vi "real time timestamp check.vi"() -> ()   [LabVIEW 2012]
uses:
  <vilib>/Utility/miscctls.llb/LVDateTimeRec.ctl
panel:
  out "epoch delta":ext format="%#_16f"
  out "unix time":ext format="%#_16f"
  out "extended precision float":ext format="%#_16f"
  out "date time rec":T1
  in  "stop":bool
  out "date/time string":string
  out "current time":timestamp
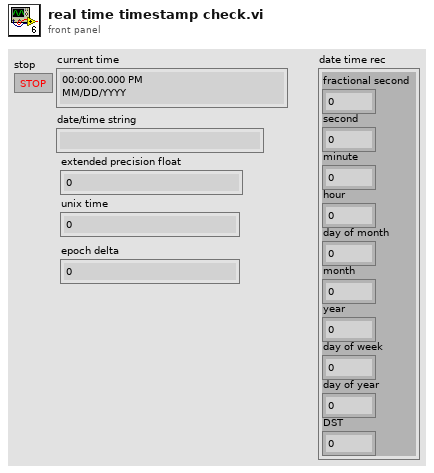
[diagram p1: front panel]
types:
  T1 = typedef "LVDateTimeRec.ctl" = cluster{"fractional second":dbl, "second":i32, "minute":i32, "hour":i32, "day of month":i32, "month":i32, "year":i32, "day of week":i32, "day of year":i32, "DST":i32}
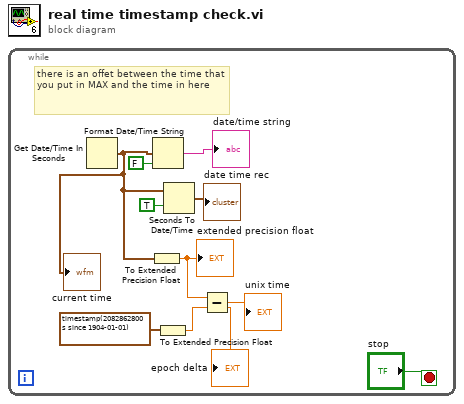
[diagram p0: block diagram]
diagram:
  n1 = while {
    stop <- "stop" stop-if-true
    # "there is an offet between the time that you put in MAX and the time in here"
    n2 = Get Date/Time In Seconds() -> (seconds since 1Jan1904=w6:timestamp)
    "current time" <- w6
    n3 = To Extended Precision Float(1:w6) -> (0:w4:ext)
    "extended precision float" <- w4
    n4 = Format Date/Time String(seconds (now)=w6, UTC format=FALSE) -> (date/time string=→"date/time string":string)  [unwired: 1 in]
    n5 = To Extended Precision Float(1:timestamp(2082862800 s since 1904-01-01)) -> (0:w2:ext)
    "epoch delta" <- w2
    n6 = Seconds To Date/Time(time stamp (now)=w6, to UTC (F)=TRUE) -> (date time rec=→"date time rec":T1)
    n7 = Subtract(x=w4, y=w2) -> (x-y=→"unix time":ext)
  }
